vi "Main Add to Queue.vi"(7 "Main Queue":T1, 11 "Main Cluster In":T3={"Main Queue"=[], "error"={"status"=FALSE, "code"=0, "source"=""}, "Camera"="", "Camera Session"="", "Image In"=refnum, "White Balance"=enum."Hold current", "Attr String"=[], "Values"=[], "VideoMode"=0, "Exposure"=50, "Reset"=FALSE} {"Exposure" min=1 max=100 scale=0.0..100.0; "VideoMode" items=["320x240 MJPG 120.10fps", "320x240 YUY2 30.00fps", "640x480 MJPG 120.10fps", "640x480 YUY2 30.00fps", "800x600 MJPG 60.00fps", "800x600 YUY2 20.00fps", "1024x768 MJPG 30.00fps", "1024x768 YUY2 6.00fps", "1280x720 MJPG 60.00fps", "1280x720 YUY2 9.00fps", "1280x1024 MJPG 30.00fps", "1280x1024 YUY2 6.00fps", "1920x1080 MJPG 30.00fps", "1920x1080 YUY2 6.00fps"]}) -> (3 "Main Cluster Out":T3={"Main Queue"=[], "error"={"status"=FALSE, "code"=0, "source"=""}, "Camera"="", "Camera Session"="", "Image In"=refnum, "White Balance"=enum."Hold current", "Attr String"=[], "Values"=[], "VideoMode"=0, "Exposure"=50, "Reset"=FALSE} {"Exposure" min=1 max=100 scale=0.0..100.0; "VideoMode" items=["320x240 MJPG 120.10fps", "320x240 YUY2 30.00fps", "640x480 MJPG 120.10fps", "640x480 YUY2 30.00fps", "800x600 MJPG 60.00fps", "800x600 YUY2 20.00fps", "1024x768 MJPG 30.00fps", "1024x768 YUY2 6.00fps", "1280x720 MJPG 60.00fps", "1280x720 YUY2 9.00fps", "1280x1024 MJPG 30.00fps", "1280x1024 YUY2 6.00fps", "1920x1080 MJPG 30.00fps", "1920x1080 YUY2 6.00fps"]})   [LabVIEW 2023]
uses:
  Ctrl's/Main Cluster.ctl
  Ctrl's/Main Queue.ctl
  Ctrl's/Main States.ctl
  <vilib>/userDefined/High Color/IMAQdx.ctl
  <vilib>/vision/Image Controls.llb/IMAQ Image.ctl
  Utilities/White Balance.ctl
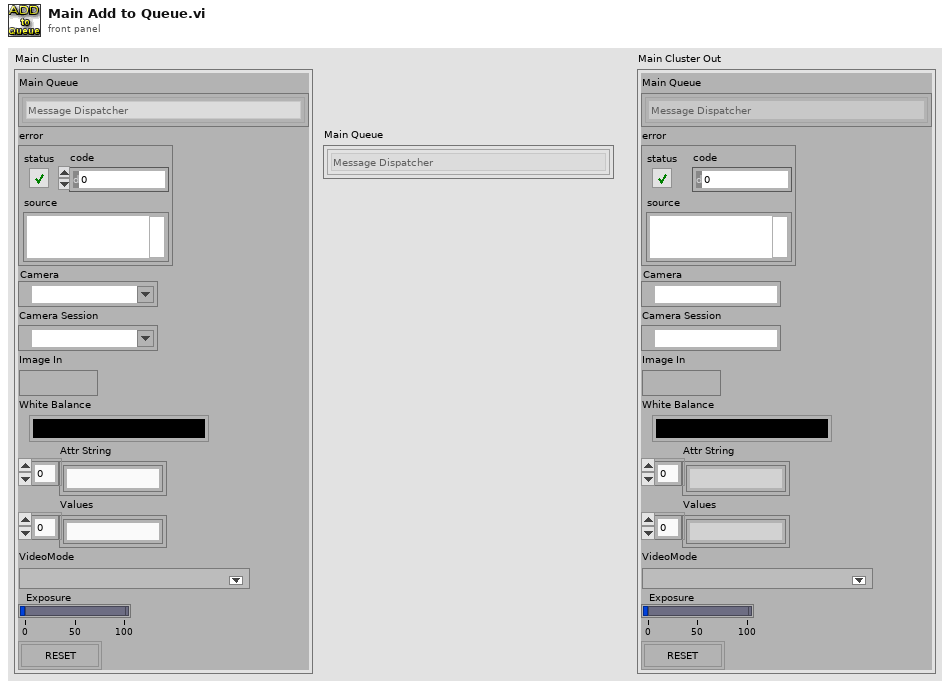
[diagram p1: front panel]
types:
  T1 = typedef "Main Queue.ctl" = T2[]
  T2 = typedef "Main States.ctl" = enum16{"Message Dispatcher", "INI", "End Session", "Camera Process Settings", "Get Contrast", "Get Gain", "Get Sharpness", "Get VideoMode", "Get Video Modes", "Save Settings", "Set Value", "Set VideoMode", "Set WB", "Setup Camera", "Start Session", "Exit"}
  T3 = typedef "Main Cluster.ctl" = cluster{"Main Queue":T1, "error":errorcluster, "Camera":T4, "Camera Session":T4, "Image In":T5, "White Balance":T6, "Attr String":string[], "Values":u16[], "VideoMode":u16, "Exposure":i32, "Reset":bool}
  T4 = typedef "IMAQdx.ctl" = refnum<k21>
  T5 = typedef "IMAQ Image.ctl" = refnum<image>
  T6 = typedef "White Balance.ctl" = enum16{"Auto", "Fixed indoor", "Fixed outdoor 1", "Fixed outdoor 2", "Fixed fluorescent 1", "Fixed fluorescent 2", "Hold current", "Custom"}
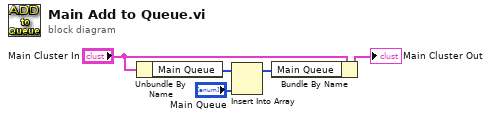
[diagram p0: block diagram]
diagram:
  n1 = Unbundle By Name("Main Cluster In") -> ("Main Queue"=w5:T1)
  n2 = Insert Into Array(array=w5, new element="Main Queue") -> (w1:T1)  [unwired: 1 in]
  n3 = Bundle By Name(cluster="Main Cluster In", "Main Queue"=w1) -> (→"Main Cluster Out":T3)
